vi "Rysowanie znacznika.vi"(9 "Znacznik na mapie":T1={"Położenie  środka"={"Pixel x"=0, "Pixel y"=0}, "Kolor "=0, "Grubość  "=2}, 10 "Zoom mapy":dbl=1.0, 11 "Mapa terenu":picture) -> (3 "Mapa z wprowadzonym znacznikiem":picture)   [LabVIEW 2012, in "Biblioteka moduł map v3.lvlib" / "Obsługa grafiki mapy.lvlib"]
doc: "Zadaniem pliku jest dorysowanie znacznika o zadanym położeniu, kolorze i grubości względem lewego górnego rogu mapy o zadanym przesunięciu i zoomie."
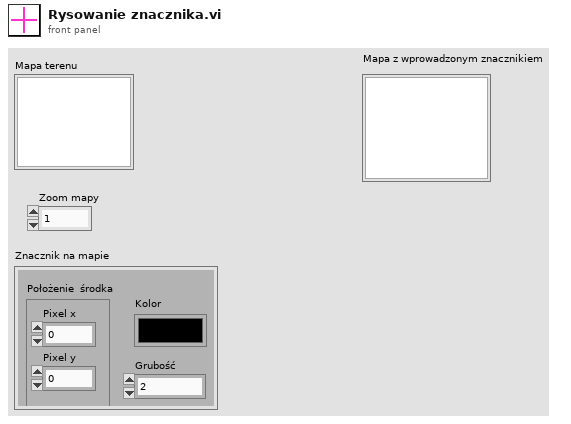
[diagram p1: front panel]
types:
  T1 = cluster{"Położenie  środka":cluster{"Pixel x":i16, "Pixel y":i16}, "Kolor ":u32, "Grubość  ":u32}
  T2 = cluster{"Width":u16, "Style":enum32{"Solid", "Dash", "Dot", "DashDot", "DashDotDot"}}
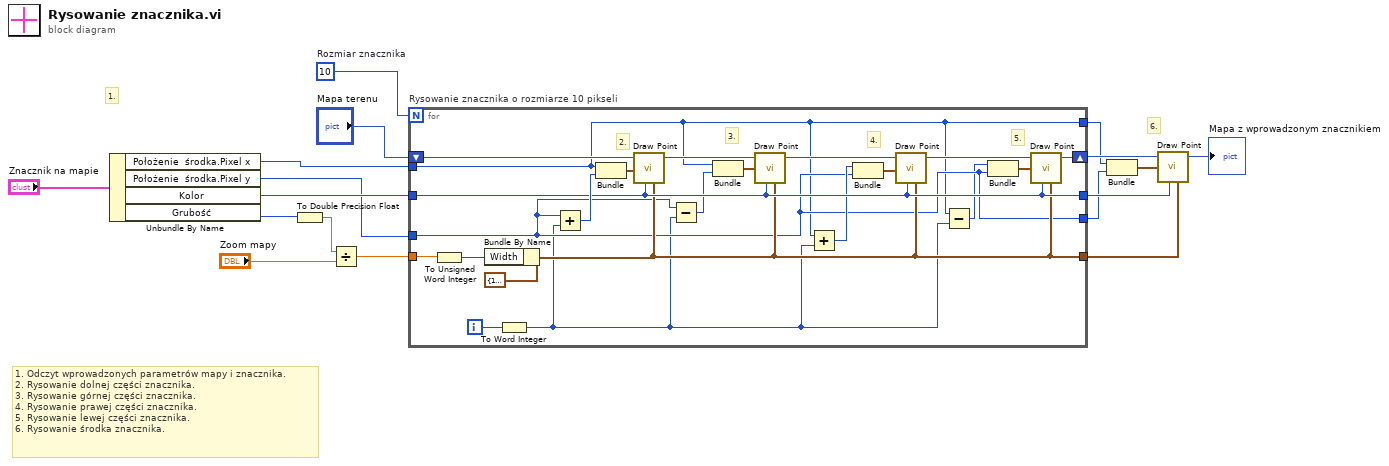
[diagram p0: block diagram]
diagram:
  w11 = 10  # Rozmiar znacznika
  # "1. Odczyt wprowadzonych parametrów mapy i znacznika.\n2. Rysowanie dolnej części znacznika.\n3. Rysowanie górnej części znacznika.\n4. Rysowanie prawej części znacznika.\n5. Rysowanie lewej części znacznika.\n6. Rysowanie środka znacznika."
  # "6."
  # "1."
  n1 = Unbundle By Name("Znacznik na mapie") -> ("Położenie  środka.Pixel x"=w2:i16, "Położenie  środka.Pixel y"=w3:i16, "Kolor"=w7:u32, "Grubość"=w5:u32)
  n2 = To Double Precision Float(number=w5) -> (double precision float=w4:dbl)
  n3 = Divide(x=w4, y="Zoom mapy") -> (x/y=w6:dbl)
  n4 = for "Rysowanie znacznika o rozmiarze 10 pikseli" {
    N: w11 -> [_]
    shift-right: [w39] -> w17
    shift-left: "Mapa terenu" -> [w38]
    tunnel: w7 -> [w33]
    tunnel: w6 -> [w19]
    tunnel: w2 -> [w23]
    tunnel: w3 -> [w25]
    tunnel: [w23] -> w16
    tunnel: [w33] -> w15
    tunnel: [w32] -> w14
    tunnel: [w25] -> w13
    i -> [w21]
    # "5."
    # "4."
    # "3."
    # "2."
    n5 = To Unsigned Word Integer(number=w19) -> (unsigned 16bit integer=w18:u16)
    n6 = Bundle By Name(cluster=T2 {"Width"=1, "Style"=enum."Solid"} ("pen"), "Width"=w18) -> (w32:T2)
    n7 = To Word Integer(number=w21) -> (16bit integer=w20:i16)
    n8 = Add(x=w25, y=w20) -> (x+y=w35:i16)
    n9 = Bundle("Pixel x"=w23, w35) -> (w34:cluster{"Pixel x":i16, i16})  [unwired: 1 in]
    n10 = call <vilib>:"Draw Point.vi"("picture"=w38, "point(x,y)"=w34, "color(black)"=w33, "pen"=w32) -> ("new picture"=w37:picture)  [unwired: 5 in]
    n11 = Subtract(x=w25, y=w20) -> (x-y=w31:i16)
    n12 = Bundle("Pixel x"=w23, w31) -> (w29:cluster{"Pixel x":i16, i16})  [unwired: 1 in]
    n13 = call <vilib>:"Draw Point.vi"("picture"=w37, "point(x,y)"=w29, "color(black)"=w33, "pen"=w32) -> ("new picture"=w30:picture)  [unwired: 5 in]
    n14 = Add(x=w23, y=w20) -> (x+y=w27:i16)
    n15 = Bundle(w27, "Pixel y"=w25) -> (w26:cluster{i16, "Pixel y":i16})  [unwired: 1 in]
    n16 = call <vilib>:"Draw Point.vi"("picture"=w30, "point(x,y)"=w26, "color(black)"=w33, "pen"=w32) -> ("new picture"=w28:picture)  [unwired: 5 in]
    n17 = Subtract(x=w23, y=w20) -> (x-y=w22:i16)
    n18 = Bundle(w22, "Pixel y"=w25) -> (w24:cluster{i16, "Pixel y":i16})  [unwired: 1 in]
    n19 = call <vilib>:"Draw Point.vi"("picture"=w28, "point(x,y)"=w24, "color(black)"=w33, "pen"=w32) -> ("new picture"=w39:picture)  [unwired: 5 in]
  }
  n20 = Bundle("Pixel x"=w16, "Pixel y"=w13) -> (w12:cluster{"Pixel x":i16, "Pixel y":i16})  [unwired: 1 in]
  n21 = call <vilib>:"Draw Point.vi"("picture"=w17, "point(x,y)"=w12, "color(black)"=w15, "pen"=w14) -> ("new picture"=→"Mapa z wprowadzonym znacznikiem":picture)  [unwired: 5 in]
